vi "getAvailableDeviceTypes.vi"(8 "error in (no error)":errorcluster, 11 "IDevice in":refnum<class "IDevice.lvclass">) -> (0 "error out":errorcluster, 2 "Device Types out":map{string, refnum<class "IDeviceType.lvclass">}(c390), 3 "IDevice out":refnum<class "IDevice.lvclass">)   [LabVIEW 2022 SP3, in "openDAQ.lvlib" / "IBaseObject.lvlib" / "IPropertyObject.lvlib" / "IComponent.lvlib" / "IFolder.lvlib" / "IDevice.lvlib" / "IDevice.lvclass"]
uses:
  <instrlib>/openDAQ/Public/Classes/IDevice/IDevice.lvclass
  <instrlib>/openDAQ/Public/Classes/IDevice/IDevice.lvclass/IDevice.ctl
  <instrlib>/openDAQ/Public/Classes/daqCoreTypes/IDict/IDict.lvclass
  <instrlib>/openDAQ/Binaries/Windows/x86/copendaq32.dll
  <instrlib>/openDAQ/Public/Classes/daqCoreTypes/IDict/Polymorphic/getValueList/getDeviceTypeValueList.vi
  <instrlib>/openDAQ/Public/Classes/IDeviceType/IDeviceType.lvclass
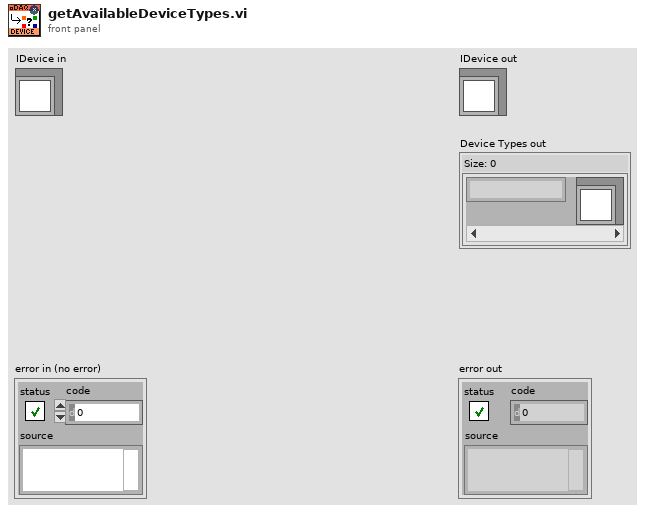
[diagram p1: front panel]
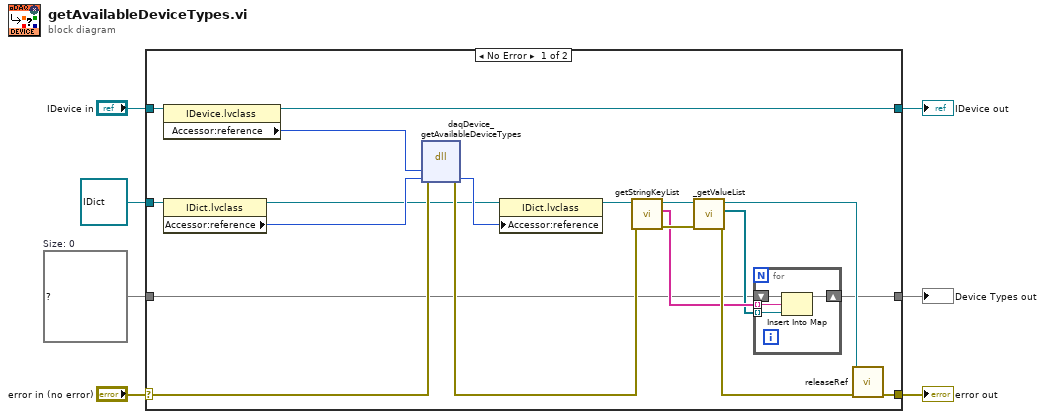
[diagram p0: block diagram]
diagram:
  w2 = map{string, refnum<class "IDeviceType.lvclass">} {}  # Size: 0
  n1 = case shown="No Error" "error in (no error)" {
    selector: "error in (no error)" -> [w23 w33]
    tunnel: [w14 w33] -> w6
    tunnel: [w22 w32] -> w4
    tunnel: "IDevice in" -> [w25 w32]
    tunnel: refnum<class "IDict.lvclass"> refnum ("openDAQ.lvlib:daqCoreTypes.lvlib:IDict.lvclass") -> [w21 _]
    tunnel: w2 -> [w10 w31]
    tunnel: [w9 w31] -> w1
    frame No Error {
      n2 = property class="IDevice.lvclass"(reference=w25) -> (reference out=w22:refnum<class "IDevice.lvclass">, "Accessor:reference"=w24:i64)  [unwired: 1 in, 1 out]
      n3 = property class="IDict.lvclass"(reference=w21) -> (reference out=w8:refnum<class "IDict.lvclass">, "Accessor:reference"=w20:i64)  [unwired: 1 in, 1 out]
      n4 = dll-call lib="C:/Program Files (x86)/National Instruments/LabVIEW 2022/instr.lib/openDAQ/Binaries/Windows/x86/copendaq*.*" fn="daqDevice_getAvailableDeviceTypes"(error in=w23, "device"=w24, "deviceTypes"=w20) -> (error out=w16:errorcluster, "deviceTypes"=w26:i64)  [unwired: 4 in, 1 out]
      n5 = property class="IDict.lvclass"(reference=w8, "Accessor:reference"=w26) -> (reference out=w19:refnum<class "IDict.lvclass">)  [unwired: 1 in, 1 out]
      n6 = call <instrlib>:"getStringKeyList.vi"("error in (no error)"=w16, "IDict in"=w19) -> ("error out"=w17:errorcluster, "Key List out"=w12:string[], "IDict out"=w18:refnum<class "IDict.lvclass">)  [unwired: 7 in]
      n7 = call-poly <instrlib>:"_getValueList.vi"("error in (no error)"=w17, "IDict in"=w18) -> ("error out"=w15:errorcluster, "Device Types out"=w11:refnum<class "IDeviceType.lvclass">[], "IDict out"=w13:refnum<class "IDict.lvclass">)  [unwired: 7 in]
      n8 = for {
        shift-right: [w27] -> w9
        shift-left: w10 -> [w30]
        tunnel: w12 -> [w29] mode=indexing
        tunnel: w11 -> [w28] mode=indexing
        n9 = Insert Into Map(map in=w30, key=w29, value=w28) -> (map out=w27:map{string, refnum<class "IDeviceType.lvclass">})  [unwired: 2 out]
      }
      n10 = call-dynamic "releaseRef.vi"("error in (no error)"=w15, "IBaseObject in"=w13) -> ("error out"=w14:errorcluster)  [unwired: 9 in]
    }
    frame Error {
    }
  }
  "error out" <- w6
  "IDevice out" <- w4
  "Device Types out" <- w1
